vi "testCheckArrSizeWithIdxArr.vi"(8 "error in (no error)":errorcluster) -> (0 "error out":errorcluster)   [LabVIEW 2016]
doc: "Test tot check the element in index array is in the spec of array size or not."
uses:
  <vilib>/addons/_JKI Toolkits/Caraya/classes/Test/Test.lvclass
  MatOper/MatOper.lvclass
  <vilib>/addons/_JKI Toolkits/Caraya/classes/Assert/Assert.lvclass
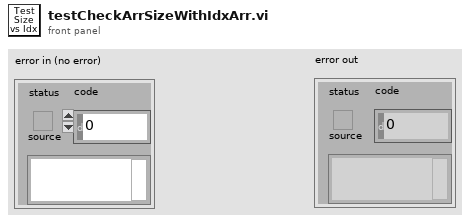
[diagram p1: front panel]
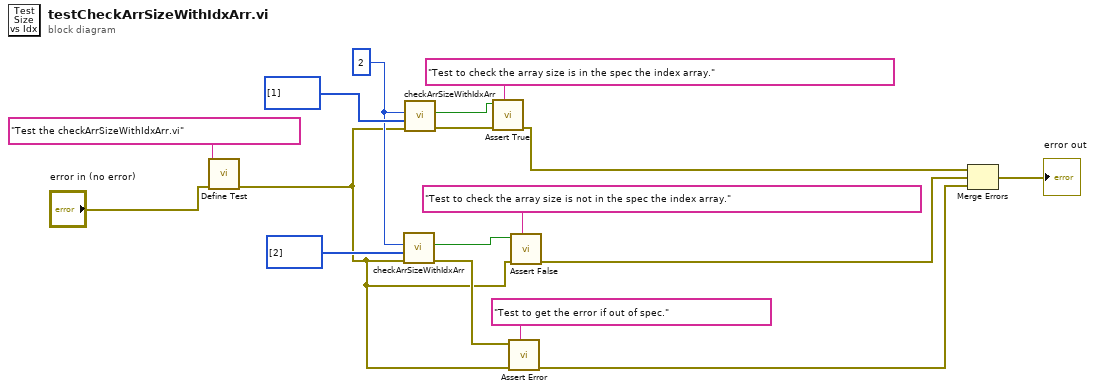
[diagram p0: block diagram]
diagram:
  w14 = 2 ("Array Size")
  n1 = call <vilib>:"Define Test.vi"("error in (no error)"="error in (no error)", "Label (VI Title)"="Test the checkArrSizeWithIdxArr.vi") -> ("error out"=w3:errorcluster)  [unwired: 9 in]
  n2 = call "checkArrSizeWithIdxArr.vi"("error in (no error)"=w3, "Idx Array"=i32[] [2], "Array Size"=w14) -> ("error out"=w5:errorcluster, "In Spec"=w6:bool)  [unwired: 6 in, 1 out]
  n3 = call "checkArrSizeWithIdxArr.vi"("error in (no error)"=w3, "Idx Array"=i32[] [1], "Array Size"=w14) -> ("error out"=w10:errorcluster, "In Spec"=w9:bool)  [unwired: 6 in, 1 out]
  n4 = call <vilib>:"Assert True.vi"("Label"="Test to check the array size is in the spec the index array.", "error in (no error)"=w10, "True?"=w9) -> ("error out"=w7:errorcluster)  [unwired: 8 in]
  n5 = call <vilib>:"Assert Error.vi"("Label"="Test to get the error if out of spec.", "error in (no error)"=w3, "Error?"=w5) -> ("error out"=w2:errorcluster)  [unwired: 8 in]
  n6 = call <vilib>:"Assert False.vi"("Label"="Test to check the array size is not in the spec the index array.", "error in (no error)"=w3, "False?"=w6) -> ("error out"=w4:errorcluster)  [unwired: 8 in]
  n7 = Merge Errors(w7, w4, w2) -> (→"error out":errorcluster)
